vi "long_test.vi"(9 "string":string="tmp\\alll.lvm", 10 "Instrument VISA in":T1={"AWG VISA"="81160A", "Oscilloscope  VISA "="Oscilloscope", "Integration Board IP"="172.16.7.43", "connection ID"=refnum, "report out"=refnum, "report file path"=path "D:/CTA/Data_test"}, 11 "error in (no error)":errorcluster) -> (3 "error out":errorcluster)   [LabVIEW 2009]
uses:
  <vilib>/Utility/NIReport.llb/NI_report.lvclass
  <vilib>/Utility/NIReport.llb/HTML/NI_HTML.lvclass
  <vilib>/Analysis/NI_AALBase.lvlib
panel:
  in  "Voltages comprobation":dbl[](array[numeric])=[0.05, 0.1, 0.2, 0.3, 0.35, 0.4, 0.45, 0.5, 0.55, 0.6, 0.7, 0.8, 0.9, 1.0, 1.2, 1.5, 1.8, 2.0]
  in  "channels":dbl[](array[numeric])=[0.0, 1.0, 2.0, 3.0, 4.0, 5.0, 6.0]
  in  "clipping":dbl[](array[numeric])=[380.0, 381.0, 396.0, 376.0, 369.0, 371.0, 333.0]
  in  "Attenuation":dbl[](array[numeric])=[1574.0, 1572.0, 1542.0, 1574.0, 1569.0, 1563.0, 1581.0]
  out "Numeric":i32
  out "atenuation":dbl[](array[numeric])=[1574.0, 1572.0, 1542.0, 1574.0, 1569.0, 1563.0, 1581.0]
  out "clipping":dbl[](array[numeric])=[380.0, 381.0, 396.0, 376.0, 369.0, 371.0, 333.0]
  out "channel":dbl[](array[numeric])=[0.0, 1.0, 2.0, 3.0, 4.0, 5.0, 6.0]
  out "XY Graph":cluster{dbl[], dbl[]}[](graph)
  out "XY Graph 2":cluster{dbl[], dbl[]}[](graph)
  out "mean value 2":dbl=8178.691389572026
  in  "stop":bool
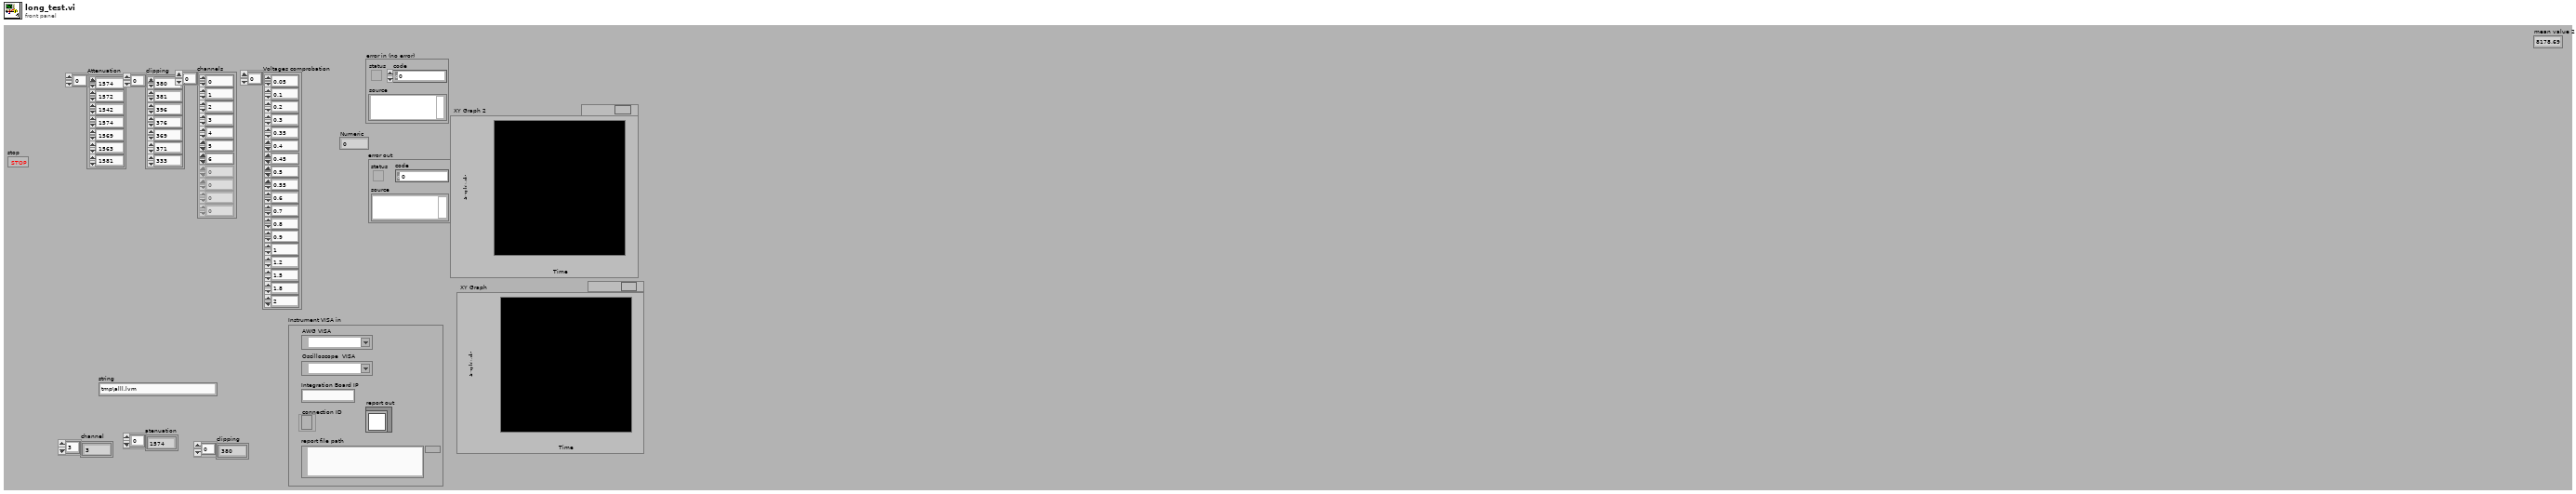
[diagram p1: front panel]
types:
  T1 = cluster{"AWG VISA":refnum<visa-resource-name>, "Oscilloscope  VISA ":refnum<visa-resource-name>, "Integration Board IP":string, "connection ID":refnum<k5>, "report out":refnum<class "NI_report.lvclass">, "report file path":path}
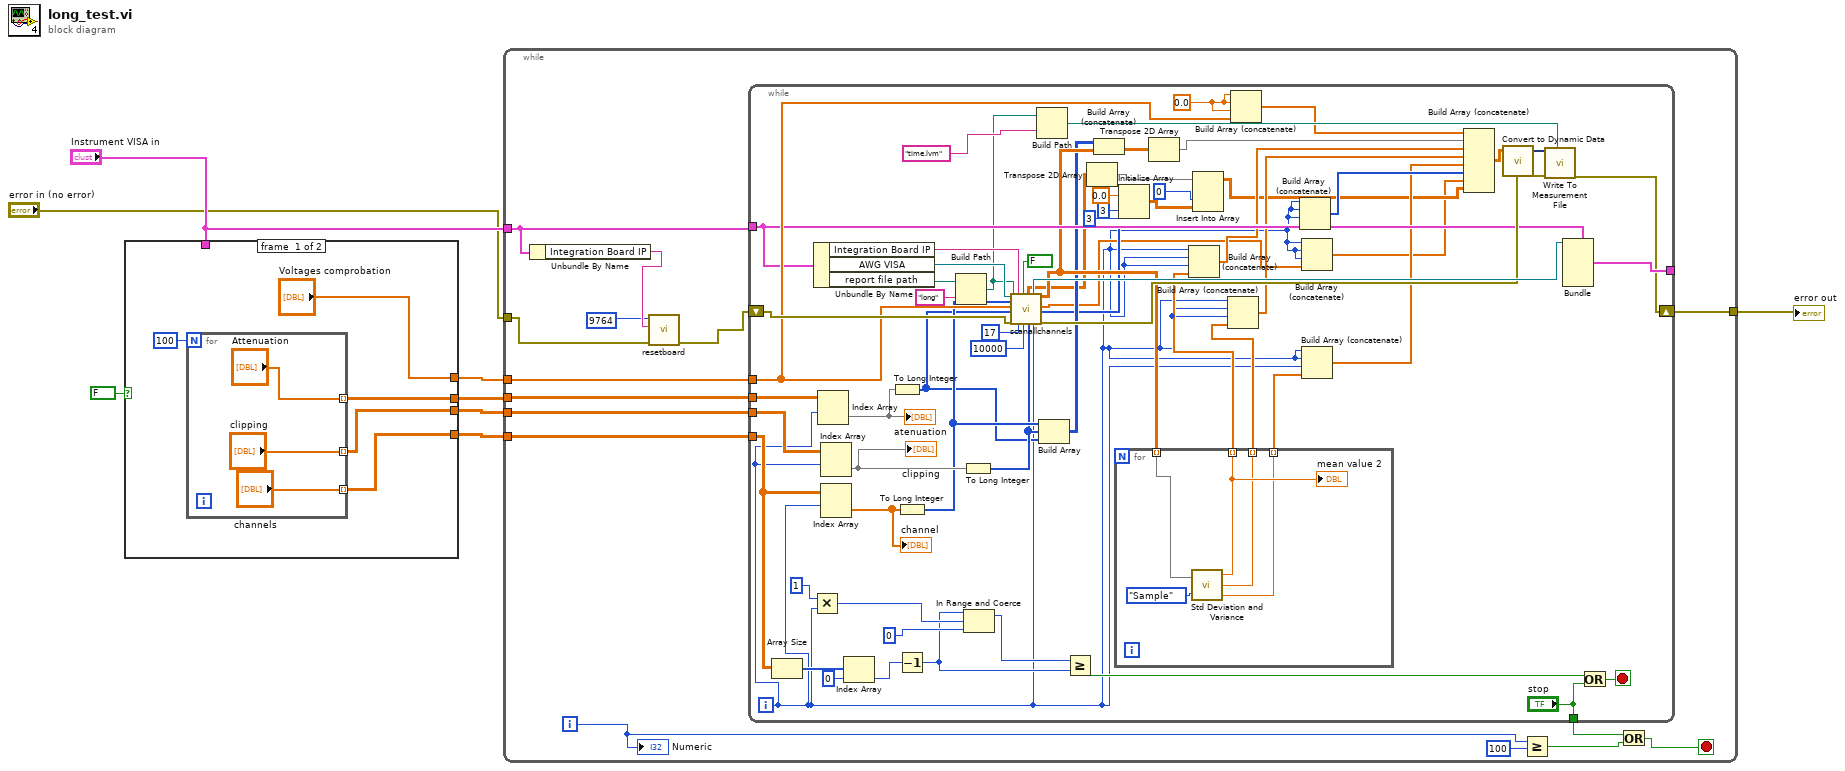
[diagram p0: block diagram]
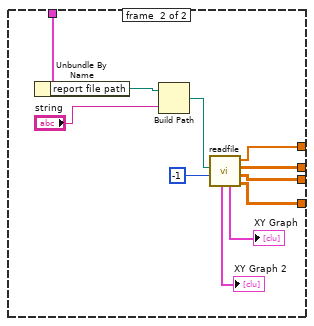
[diagram p2: hidden frame]
diagram:
  n1 = case shown="False" FALSE {
    tunnel: ["Voltages comprobation" w24] -> w8
    tunnel: "Instrument VISA in" -> [_ w23]
    tunnel: [w11 w22] -> w6
    tunnel: [w12 w21] -> w5
    tunnel: [w13 w20] -> w4
    frame #0 {
      n2 = for {
        N: 100 -> [_]
        tunnel: ["Attenuation"] -> w13 mode=indexing
        tunnel: ["clipping"] -> w12 mode=indexing
        tunnel: ["channels"] -> w11 mode=indexing
      }
    }
    frame #1 {
      n3 = Unbundle By Name(w23) -> ("report file path"=w19:path)
      n4 = Build Path(base path=w19, name or relative path="string") -> (appended path=w18:path)
      n5 = call "readfile.vi"("count"=-1, "file (use dialog)"=w18) -> ("channels"=w22:dbl[][], "clipping"=w21:dbl[][], "attenuator"=w20:dbl[][], "voltage"=w24:dbl[], "XY Graph"=→"XY Graph":cluster{dbl[], dbl[]}[], "XY Graph 2"=→"XY Graph 2":cluster{dbl[], dbl[]}[])  [unwired: 4 in]
    }
  }
  n6 = while {
    tunnel: w8 -> [w42]
    tunnel: "Instrument VISA in" -> [w35]
    tunnel: w6 -> [w41]
    tunnel: w5 -> [w40]
    tunnel: w4 -> [w39]
    tunnel: [w34] -> w3
    tunnel: "error in (no error)" -> [w33]
    i -> [w28]
    stop <- w31 stop-if-true
    n7 = Unbundle By Name(w35) -> ("Integration Board IP"=w38:string)
    n8 = call "resetboard.vi"("error in (no error)"=w33, "address"=w38, "remote port or service name"=u16 9764) -> ("error out"=w37:errorcluster)  [unwired: 7 in, 1 out]
    n9 = while {
      tunnel: w42 -> [w95]
      tunnel: w35 -> [w92]
      tunnel: [w93] -> _
      shift-right: [w89] -> w34
      shift-left: w37 -> [w99]
      tunnel: w41 -> [w86]
      tunnel: w40 -> [w87]
      tunnel: w39 -> [w88]
      tunnel: ["stop"] -> w30
      i -> [w43]
      stop <- w83 stop-if-true
      w100 = 0.0 ("element")
      n10 = Array Size(array=w86) -> (size(s)=w85:i32[])
      n11 = Multiply(x=1 ("index"), y=w43) -> (x*y=w57:i32)
      n12 = Unbundle By Name(w92) -> ("Integration Board IP"=w91:string, "AWG VISA"=w90:refnum<visa-resource-name>, "report file path"=w78:path)
      n13 = Index Array(array=w88, index (row)=w43) -> (element=w79:dbl[])  [unwired: 1 in]
      "atenuation" <- w79
      n14 = Index Array(array=w87, index (row)=w43) -> (element=w81:dbl[])  [unwired: 1 in]
      "clipping" <- w81
      n15 = Index Array(array=w86, index (row)=w43) -> (element=w80:dbl[])  [unwired: 1 in]
      "channel" <- w80
      n16 = Index Array(array=w85, index=0) -> (element=w58:i32)
      n17 = To Long Integer(number=w79) -> (32bit integer=w72:i32[])
      n18 = To Long Integer(number=w80) -> (32bit integer=w74:i32[])
      n19 = Decrement(x=w58) -> (x-1=w56:i32)
      n20 = Build Path(base path=w78, name or relative path="long") -> (appended path=w77:path)
      n21 = To Long Integer(number=w81) -> (32bit integer=w73:i32[])
      n22 = In Range and Coerce(upper limit=w56, x=w57, lower limit=0) -> (coerced(x)=w55:i32)  [unwired: 1 out]
      n23 = call "scanallchannels.vi"("VISA resource name in"=w90, "nm ch"=w74, "Voltages values"=w95, "Init ch value"=w72, "base path"=w77, "error in"=w99, "Integration Board IP"=w91, "L1 Address"=17, "Save test data"=FALSE, "Ch burst"=10000, "vclip"=w73, "Delay"=w43) -> ("Amp&width"=w54:dbl[][], "VISA resource name out"=w104:refnum<visa-resource-name>, "Array"=w71:dbl[][], "temperatura"=w45:dbl[], "time"=w67:u32[], "error out"=w102:errorcluster)  [unwired: 1 in, 1 out]
      n24 = Build Path(base path=w77, name or relative path="time.lvm" ("string")) -> (appended path=w106:path)
      n25 = Build Array(w74, w73, w72) -> (w70:i32[][])
      n26 = Greater Or Equal?(x=w55, y=w56) -> (x >= y?=w82:bool)
      n27 = Transpose 2D Array(2D array=w54) -> (transposed array=w52:dbl[][])
      n28 = Build Array (concatenate)(w70, w71) -> (w69:dbl[][])
      n29 = for {
        tunnel: w71 -> [w111] mode=indexing
        tunnel: [w109] -> w65 mode=indexing
        tunnel: [w108] -> w64 mode=indexing
        tunnel: [w107] -> w62 mode=indexing
        n30 = call <vilib>:"Std Deviation and Variance.vi"("X"=w111, "Weighting (Sample)"=enum16{"Sample", "Population"}."Sample") -> ("mean"=w109:dbl, "standard deviation"=w108:dbl, "variance"=w107:dbl)
        "mean value 2" <- w109
      }
      n31 = Initialize Array(0.0 ("element"), 3 ("dimension size"), 3 ("dimension size")) -> (w51:dbl[][])
      n32 = Transpose 2D Array(2D array=w69) -> (transposed array=w105:dbl[][])
      n33 = Build Array (concatenate)(w43, w43, w43, w65) -> (w66:dbl[])
      n34 = Insert Into Array(array=w52, index (col)=0 ("disabled index (col)"), new element=w51) -> (w46:dbl[][])  [unwired: 1 in]
      n35 = Build Array (concatenate)(w43, w43, w43, w64) -> (w63:dbl[])
      n36 = Build Array (concatenate)(w100, w100, w100, w95) -> (w53:dbl[])
      n37 = Build Array (concatenate)(w43, w43, w43, w67) -> (w68:u32[])
      n38 = Build Array (concatenate)(w43, w43, w43, w45) -> (w44:dbl[])
      n39 = Build Array (concatenate)(w43, w43, w43, w62) -> (w61:dbl[])
      n40 = Build Array (concatenate)(w53, w105, w66, w63, w61, w68, w44, w46) -> (w103:dbl[][])
      n41 = call "Convert to Dynamic Data"("2D Array"=w103) -> ("Dynamic Data Type"=w101:dynamicdata)  [unwired: 3 in]
      n42 = call "Write To Measurement File"("Signals"=w101, "error in (no error)"=w102, "Filename"=w106) -> ("error out"=w89:errorcluster)  [unwired: 14 in, 2 out]
      n43 = Bundle(cluster=w92, "AWG VISA"=w104) -> (w93:T1)  [unwired: 5 in]
      n44 = Or(x=w82, y="stop") -> (x .or. y?=w83:bool)
    }
    n45 = Greater Or Equal?(x=w28, y=100) -> (x >= y?=w29:bool)
    n46 = Or(x=w30, y=w29) -> (x .or. y?=w31:bool)
    "Numeric" <- w28
  }
  "error out" <- w3
